vi "3-4.vi"() -> ()   [LabVIEW 2017]
panel:
  out "长度":i32
  in  "数值2":dbl
  out "显示":string
  in  "输入3":string
  in  "输入1":string
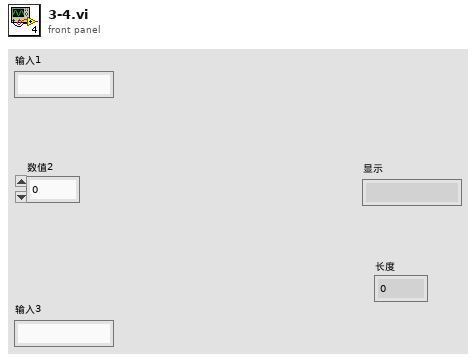
[diagram p1: front panel]
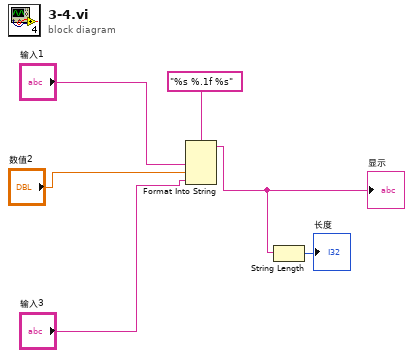
[diagram p0: block diagram]
diagram:
  n1 = Format Into String(format string="%s %.1f %s" ("格式字符串"), "输入1", "数值2", "输入3") -> (resulting string=w1:string)  [unwired: 2 in, 1 out]
  "显示" <- w1
  n2 = String Length(string=w1) -> (length=→"长度":i32)
